vi "AI Read Value.vi"(7 "ADC #":T1=-1, 8 "error in (no error)":errorcluster, 11 "Session in":refnum<class "Session.lvclass">) -> (0 "error out":errorcluster, 2 "Value":T2, 3 "Session out":refnum<class "Session.lvclass">)   [LabVIEW 2024, in "CTI.lvlib" / "Session.lvclass"]
doc: "Returns the Raw ADC value for the specified analog input. The ADC must first have been configured by calling <b>Configure AI.vi</b>.\n\nThe returned raw ADC value will relative to the device's analog reference voltage and would typically need to be scaled to a voltage or engineering units for proper usage."
uses:
  Session.lvclass
  Raw ADC.ctl
  ADC Number.ctl
  DeviceComms/DeviceComms.lvclass
  CTI.lvlib
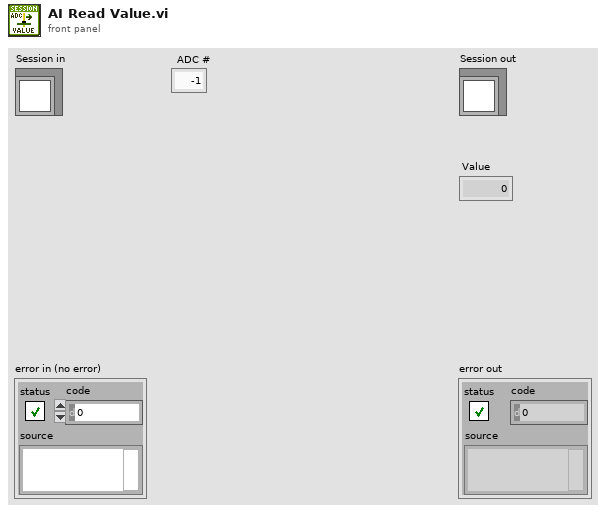
[diagram p1: front panel]
types:
  T1 = typedef "CTI.lvlib/ADC Number.ctl" = i8
  T2 = typedef "CTI.lvlib/Raw ADC.ctl" = u16
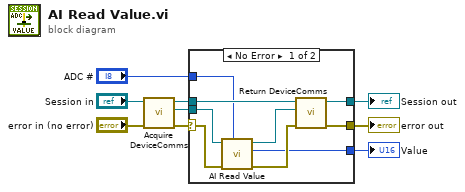
[diagram p0: block diagram]
diagram:
  n1 = call "Acquire DeviceComms.vi"("error in (no error)"="error in (no error)", "Session in"="Session in") -> ("error out"=w8:errorcluster, "DeviceComms"=w7:refnum<class "DeviceComms.lvclass">, "Session out"=w9:refnum<class "Session.lvclass">)  [unwired: 7 in]
  n2 = case shown="No Error" w8 {
    selector: w8 -> [w10 w20]
    tunnel: w9 -> [w17 w19]
    tunnel: w7 -> [w18 _]
    tunnel: [w14 w19] -> w3
    tunnel: [w13 w20] -> w4
    tunnel: "ADC #" -> [w12 _]
    tunnel: [w11 _] -> w5
    frame No Error {
      n3 = call-dynamic "AI Read Value.vi"("ADC #"=w12, "error in (no error)"=w10, "DeviceComms in"=w18) -> ("error out"=w15:errorcluster, "Value"=w11:T2, "DeviceComms out"=w16:refnum<class "DeviceComms.lvclass">)  [unwired: 6 in]
      n4 = call "Return DeviceComms.vi"("error in (no error)"=w15, "DeviceComms"=w16, "Session in"=w17) -> ("error out"=w13:errorcluster, "Session out"=w14:refnum<class "Session.lvclass">)  [unwired: 7 in]
    }
    frame Error {
    }
  }
  "error out" <- w4
  "Session out" <- w3
  "Value" <- w5
